vi "Get IO Types.vi"(8 "error in (no error)":errorcluster, 11 "TestBlock in":refnum<class "TestBlock.lvclass">) -> (0 "error out":errorcluster, 2 "Types":refnum<class "Type Descriptor.lvclass">[](array[class]), 3 "TestBlock out":refnum<class "TestBlock.lvclass">)   [LabVIEW 2020, in "TestBlock.lvclass"]
uses:
  TestBlock.lvclass
  TestBlock.lvclass/TestBlock.ctl
  c9e03f35-803e-4603-b9f9-f1dc9a2d3a48.vi
  db941595-8d40-4aa8-a54c-6f1eda7cda3e.vi
  5809c432-f075-41f7-b429-66f414819210.vi
  1130a341-6a03-4352-a2f2-d1642be82d7f.vi
  0d8caef8-b2d4-49a5-b055-bc22df2db35f.vi
  Parallel Block/DBL Wfm.ctl
  Parallel Block/Parallel Block.lvlib
  Parallel Block/Type Mode.ctl
  Parallel Block/Type Descriptor/Type Descriptor.lvclass
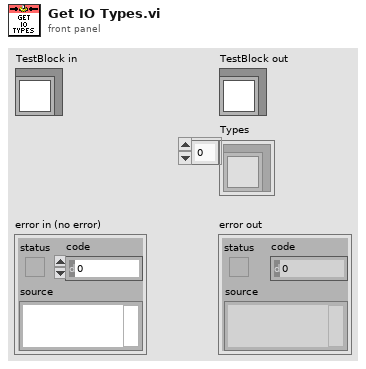
[diagram p1: front panel]
types:
  T1 = typedef "Parallel Block.lvlib/Type Mode.ctl" = enum16{"Output", "Single - Strict", "Single - Coerced", "Stream"}
  T2 = typedef "Parallel Block.lvlib/DBL Wfm.ctl" = cluster{"x0":dbl, "dx":dbl, "y":dbl[]}
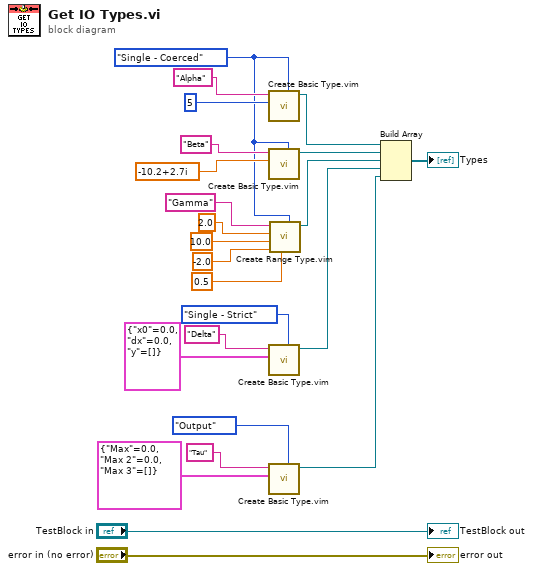
[diagram p0: block diagram]
diagram:
  w2 = Type_Mode."Single - Coerced" ("Type Mode")
  n1 = call "Create Basic Type.vim"("Type Mode"=w2, "Type & Default"=5, "Name"="Alpha") -> ("Type Descriptor"=w17:refnum<class "Type Descriptor.lvclass">)  [unwired: 8 in]
  n2 = call "Create Basic Type.vim"("Type Mode"=w2, "Type & Default"=cdb -10.2+2.7i, "Name"="Beta") -> ("Type Descriptor"=w18:refnum<class "Type Descriptor.lvclass">)  [unwired: 8 in]
  n3 = call "Create Basic Type.vim"("Type Mode"=Type_Mode."Single - Strict", "Type & Default"=T2 {"x0"=0.0, "dx"=0.0, "y"=[]} ("DBL Wfm"), "Name"="Delta") -> ("Type Descriptor"=w10:refnum<class "Type Descriptor.lvclass">)  [unwired: 8 in]
  n4 = call "Create Basic Type.vim"("Type Mode"=Type_Mode."Output", "Type & Default"=cluster{"Max":dbl, "Max 2":dbl, "Max 3":cdb[]} {"Max"=0.0, "Max 2"=0.0, "Max 3"=[]}, "Name"="Tau") -> ("Type Descriptor"=w4:refnum<class "Type Descriptor.lvclass">)  [unwired: 8 in]
  n5 = call "Create Range Type.vim"("Type Mode"=w2, "Step"=0.5, "Min"=-2.0, "Max"=10.0, "Type & Default"=2.0, "Name"="Gamma") -> ("Type Descriptor"=w12:refnum<class "Type Descriptor.lvclass">)  [unwired: 5 in]
  n6 = Build Array(w17, w18, w12, w10, w4) -> (→"Types":refnum<class "Type Descriptor.lvclass">[])
  "error out" <- "error in (no error)"
  "TestBlock out" <- "TestBlock in"
